vi "Publish DI.vi"(8 "error in":errorcluster, 10 "DI Data":bool[](array[boolean]), 11 "BNT_DAQmx-MCSV in":refnum<class "BNT_DAQmx-MCSV.lvclass">) -> (0 "error out":errorcluster, 3 "BNT_DAQmx-MCSV out":refnum<class "BNT_DAQmx-MCSV.lvclass">)   [LabVIEW 2021, in "BNT_DAQmx.lvlib" / "BNT_DAQmx-MCSV.lvclass"]
doc: "Publish digital input values if changed."
uses:
  BNT_DAQmx-MCSV.lvclass
  BNT_DAQmx-MCSV.lvclass/BNT_DAQmx-MCSV.ctl
  CSPP_Core/Classes/CSPP_ProcessVariables/PVConnection/PVConnection.lvclass/PVConnection.ctl
  CSPP_Core/Classes/CSPP_ProcessVariables/ProcessVariable/PV.lvclass/PV.ctl
  CSPP_Core/Classes/CSPP_ProcessVariables/ProcessVariable/Write Data.vi
  CSPP_Core/Classes/CSPP_ProcessVariables/ProcessVariable/Write Error.vi
  CSPP_Core/Classes/CSPP_ProcessVariables/ProcessVariable/Write Quality.vi
  CSPP_Core/Classes/CSPP_ProcessVariables/ProcessVariable/Write status.vi
  CSPP_Core/Classes/CSPP_ProcessVariables/ProcessVariable/Write Timestamp.vi
  CSPP_Core/Classes/CSPP_ProcessVariables/ProcessVariable/PV.lvclass
  CSPP_Core/Classes/CSPP_ProcessVariables/PVConnection/PVConnection.lvclass
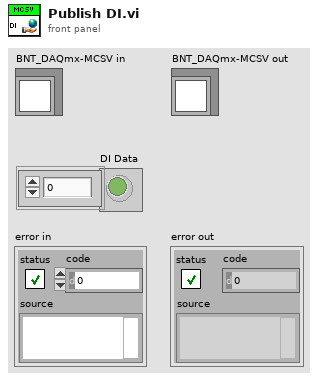
[diagram p1: front panel]
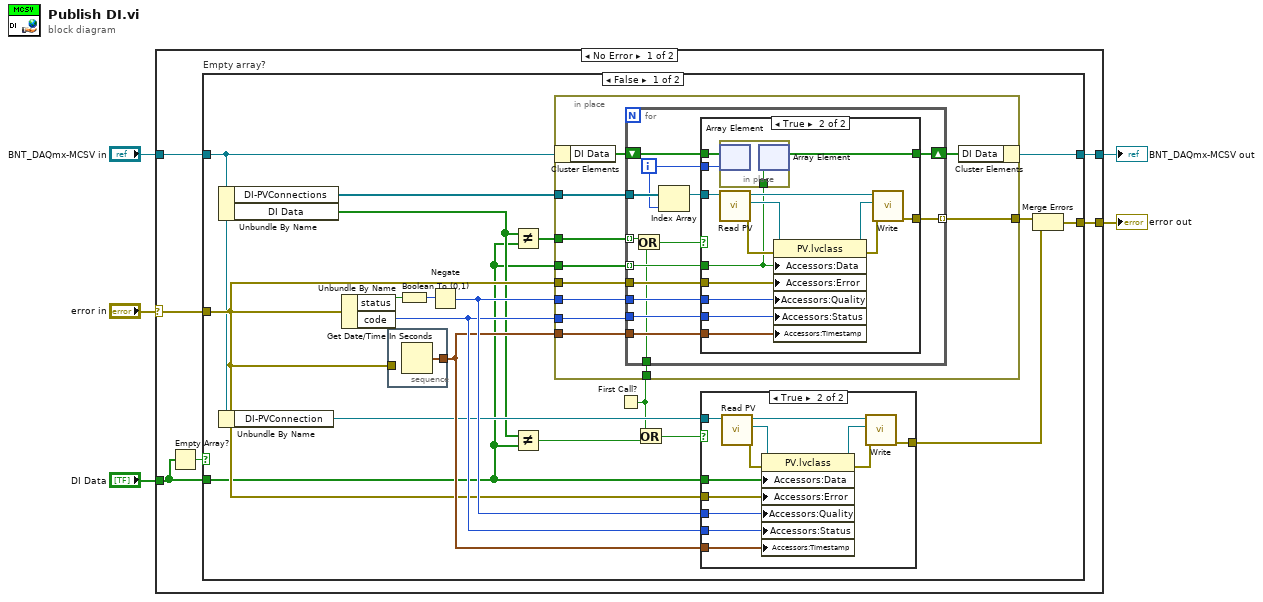
[diagram p0: block diagram]
diagram:
  n1 = case shown="No Error" "error in" {
    selector: "error in" -> [w11 w91]
    tunnel: [w10 w91] -> w4
    tunnel: [w8 w90] -> w2
    tunnel: "BNT_DAQmx-MCSV in" -> [w9 w90]
    tunnel: "DI Data" -> [w6 _]
    frame No Error {
      n2 = Empty Array?(array=w6) -> (empty?=w7:bool)
      n3 = case "Empty array?" shown="False" w7 {
        tunnel: w11 -> [w23 w88]
        tunnel: [w21 w88] -> w10
        tunnel: w9 -> [w16 w89]
        tunnel: [w15 w89] -> w8
        tunnel: w6 -> [w13 _]
        frame False {
          n4 = Unbundle By Name(w16) -> ("DI-PVConnections"=w22:refnum<class "PVConnection.lvclass">[], "DI Data"=w18:bool[])
          n5 = Unbundle By Name(w16) -> ("DI-PVConnection"=w20:refnum<class "PVConnection.lvclass">)
          n6 = Unbundle By Name(w23) -> ("status"=w29:bool, "code"=w26:i32)
          n7 = stacked-sequence {
            tunnel: [w31] -> w25
            tunnel: w23 -> [_]
            frame #0 {
              n8 = Get Date/Time In Seconds() -> (seconds since 1Jan1904=w31:timestamp)
            }
          }
          n9 = Boolean To (0,1)(Boolean=w29) -> (0, 1=w28:i16)
          n10 = Negate(x=w28) -> (-x=w27:i16)
          n11 = Not Equal?(x=w18, y=w13) -> (x != y?=w19:bool[])
          n12 = Not Equal?(x=w18, y=w13) -> (x != y?=w17:bool)
          n13 = First Call?() -> (First Call?: T/F=w12:bool)
          n14 = in-place {
            in-place-border: [w42] -> w30
            in-place-border: w27 -> [w41]
            in-place-border: w26 -> [w40]
            in-place-border: w25 -> [w39]
            in-place-border: w23 -> [w38]
            in-place-border: w22 -> [w37]
            in-place-border: w13 -> [w36]
            in-place-border: w19 -> [w35]
            in-place-border: w12 -> [w32]
            n15 = in-place-cluster #1(w16) -> ("DI Data"=w34:bool[])
            n16 = for {
              tunnel: w37 -> [w50]
              tunnel: w36 -> [w56] mode=indexing
              tunnel: w38 -> [w55]
              tunnel: [w54] -> w42 mode=indexing
              tunnel: w41 -> [w53]
              tunnel: w40 -> [w52]
              tunnel: w39 -> [w51]
              tunnel: w35 -> [w49] mode=indexing
              shift-right: [w47] -> w33
              shift-left: w34 -> [w48]
              tunnel: w32 -> [w45]
              i -> [w43]
              n17 = Or(x=w49, y=w45) -> (x .or. y?=w46:bool)
              n18 = Index Array(array=w50, index=w43) -> (element=w44:refnum<class "PVConnection.lvclass">)
              n19 = case shown="True" w46 {
                tunnel: w56 -> [_ w60]
                tunnel: w55 -> [w58 w73]
                tunnel: [w58 w70] -> w54
                tunnel: w53 -> [_ w69]
                tunnel: w52 -> [_ w68]
                tunnel: w51 -> [_ w67]
                tunnel: w44 -> [_ w66]
                tunnel: w43 -> [_ w62]
                tunnel: w48 -> [w57 w61]
                tunnel: [w57 w59] -> w47
                frame False {
                }
                frame True {
                  n20 = in-place {
                    in-place-border: w60 -> [w74]
                    n21 = in-place-array #2(w61, w62) -> ()  [unwired: 1 out]
                    n22 = in-place-array #2(w74) -> (w59:bool[])  [unwired: 1 out]
                  }
                  n23 = call "Read PV.vi"("PVConnection in"=w66) -> ("error out"=w63:errorcluster, "PV"=w64:refnum<class "PV.lvclass">, "PVConnection out"=w65:refnum<class "PVConnection.lvclass">)  [unwired: 8 in]
                  n24 = property class="PV.lvclass"(reference=w64, error in=w63, "Accessors:Data"=w60, "Accessors:Error"=w73, "Accessors:Quality"=w69, "Accessors:Status"=w68, "Accessors:Timestamp"=w67) -> (reference out=w72:refnum<class "PV.lvclass">, error out=w71:errorcluster)
                  n25 = call "Write.vi"("error in (no error)"=w71, "PV"=w72, "PVConnection in"=w65) -> ("error out"=w70:errorcluster)  [unwired: 6 in, 2 out]
                }
              }
            }
            n26 = in-place-cluster #1("DI Data"=w33) -> (w15:refnum<class "BNT_DAQmx-MCSV.lvclass">)
          }
          n27 = Or(x=w12, y=w17) -> (x .or. y?=w14:bool)
          n28 = case shown="True" w14 {
            tunnel: w27 -> [_ w82]
            tunnel: w26 -> [_ w81]
            tunnel: w25 -> [_ w80]
            tunnel: [w75 w79] -> w24
            tunnel: w23 -> [w75 w78]
            tunnel: w20 -> [_ w77]
            tunnel: w13 -> [_ w76]
            frame False {
            }
            frame True {
              n29 = call "Read PV.vi"("PVConnection in"=w77) -> ("error out"=w83:errorcluster, "PV"=w84:refnum<class "PV.lvclass">, "PVConnection out"=w85:refnum<class "PVConnection.lvclass">)  [unwired: 8 in]
              n30 = property class="PV.lvclass"(reference=w84, error in=w83, "Accessors:Data"=w76, "Accessors:Error"=w78, "Accessors:Quality"=w82, "Accessors:Status"=w81, "Accessors:Timestamp"=w80) -> (reference out=w87:refnum<class "PV.lvclass">, error out=w86:errorcluster)
              n31 = call "Write.vi"("error in (no error)"=w86, "PV"=w87, "PVConnection in"=w85) -> ("error out"=w79:errorcluster)  [unwired: 6 in, 2 out]
            }
          }
          n32 = Merge Errors(w30, w24) -> (w21:errorcluster)
        }
        frame True {
        }
      }
    }
    frame Error {
    }
  }
  "error out" <- w4
  "BNT_DAQmx-MCSV out" <- w2
